vi "Run.vi"(8 "error in (no error)":errorcluster, 11 "VideoMux in":refnum<class "VideoMux.lvclass">) -> (0 "error out":errorcluster, 3 "VideoMux out":refnum<class "VideoMux.lvclass">)   [LabVIEW 2022 SP3, in "VideoMux.lvlib" / "VideoMux.lvclass"]
uses:
  VideoMux.lvclass
  VideoMux.lvclass/VideoMux.ctl
  <vilib>/IlluminatedG/IG HTTP Server/HTTP Server/Server/Server.lvclass
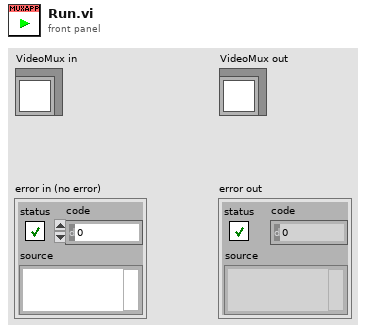
[diagram p1: front panel]
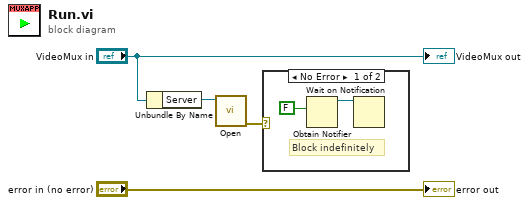
[diagram p0: block diagram]
diagram:
  n1 = Unbundle By Name("VideoMux in") -> ("Server"=w2:refnum<class "Server.lvclass">)
  n2 = call <vilib>:"Open.vi"("Server in"=w2) -> ("error out"=w1:errorcluster)  [unwired: 9 in, 1 out]
  n3 = case shown="No Error" w1 {
    frame No Error {
      # "Block indefinitely"
      n4 = Obtain Notifier(notification data type=FALSE) -> (notifier out=w6:refnum<notifier>)  [unwired: 3 in, 2 out]
      n5 = Wait on Notification(notifier=w6) -> ()  [unwired: 3 in, 4 out]
    }
    frame Error {
    }
  }
  "error out" <- "error in (no error)"
  "VideoMux out" <- "VideoMux in"
